vi "Power Change.vi"(11 "Array":dbl[](array[numeric])) -> (3 "Reactor Power (W)":dbl)   [LabVIEW 2019]
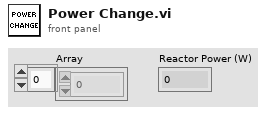
[diagram p1: front panel]
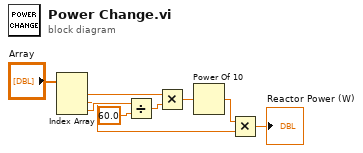
[diagram p0: block diagram]
diagram:
  n1 = Index Array(array="Array") -> (element #1=w7:dbl, element #2=w8:dbl, element #3=w9:dbl)  [unwired: 3 in]
  n2 = Divide(x=w9, y=60.0) -> (x/y=w2:dbl)
  n3 = Multiply(x=w7, y=w2) -> (x*y=w3:dbl)
  n4 = Power Of 10(x=w3) -> (10^x=w4:dbl)
  n5 = Multiply(x=w4, y=w8) -> (x*y=→"Reactor Power (W)":dbl)
